vi "Subscribe to UI Launched.vi"(8 "error in":errorcluster, 9 "Message":refnum<class "Message.lvclass">, 10 "Enqueuer":refnum<class "Message Enqueuer.lvclass">, 11 "Flex UI (Actor) in":refnum<class "Flex UI (Actor).lvclass">) -> (0 "error out":errorcluster, 3 "Flex UI (Actor) out":refnum<class "Flex UI (Actor).lvclass">)   [LabVIEW 2016, in "Flex UI (Parent Actor).lvlib" / "Flex UI (Actor).lvclass"]
uses:
  Flex UI (Actor).lvclass
  <vilib>/ActorFramework/Message/Message.lvclass
  <vilib>/ActorFramework/Message Enqueuer/Message Enqueuer.lvclass
  Flex UI (Actor).lvclass/Flex UI (Actor).ctl
  <vilib>/East West Architects/MVC Subscription/Subscription/MVC Subscription.lvclass
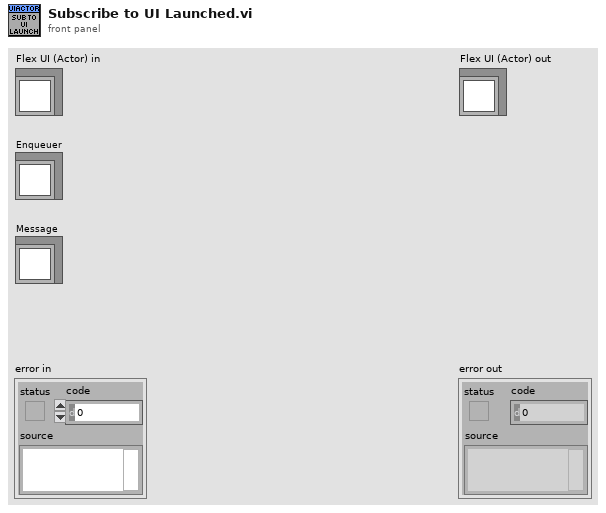
[diagram p1: front panel]
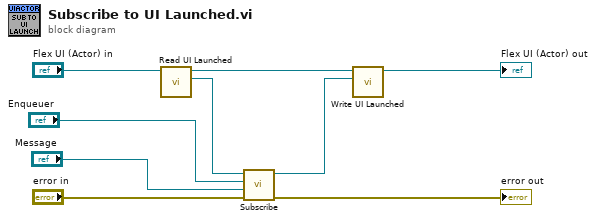
[diagram p0: block diagram]
diagram:
  n1 = call "Read UI Launched.vi"("Flex UI (Actor) in"="Flex UI (Actor) in") -> ("Subscriptions.UI Launched"=w3:refnum<class "MVC Subscription.lvclass">, "Flex UI (Actor) out"=w8:refnum<class "Flex UI (Actor).lvclass">)  [unwired: 9 in]
  n2 = call <vilib>:"Subscribe.vi"("error in"="error in", "Message"="Message", "Enqueuer"="Enqueuer", "MVC Subscription in"=w3) -> ("error out"=→"error out":errorcluster, "MVC Subscription out"=w4:refnum<class "MVC Subscription.lvclass">)  [unwired: 6 in]
  n3 = call "Write UI Launched.vi"("Subscriptions.UI Launched"=w4, "Flex UI (Actor) in"=w8) -> ("Flex UI (Actor) out"=→"Flex UI (Actor) out":refnum<class "Flex UI (Actor).lvclass">)  [unwired: 9 in]
